vi "set_iterations_per_pixel.vi"(8 "error in (no error)":errorcluster, 10 "iterations per pixel":i32, 11 "FPGAWrapperAN110607Galvo in":refnum<class "FPGAWrapperAN110607Galvo.lvclass">) -> (0 "error out":errorcluster, 3 "FPGAWrapperAN110607Galvo out":refnum<class "FPGAWrapperAN110607Galvo.lvclass">)   [LabVIEW 2010, in "FPGAWrapperAN110607Galvo.lvclass"]
uses:
  FPGAWrapperAN110607Galvo.lvclass
  <vilib>/rvi/interface/nirviReadWriteControl/nirviReadWriteControl.xnode
  FPGA_VI_ref.ctl
  <vilib>/rvi/interface/common/niFpgaNodeNameForErrorReporting.ctl
  <vilib>/rvi/errors/niLvFpgaWhatHappensToTopLevelVI.ctl
  <vilib>/Utility/error.llb/Error Cluster From Error Code.vi
  <vilib>/rvi/errors/niLvFpgaAdjustHostInterfaceError.vi
  NiFpgaLv.dll
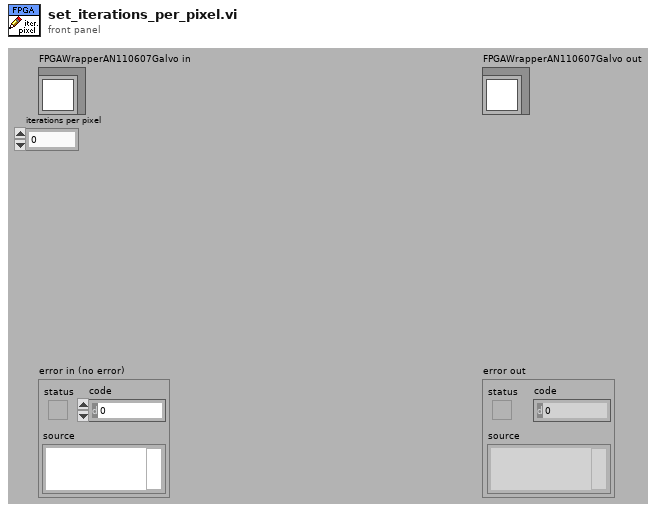
[diagram p1: front panel]
types:
  T1 = typedef "niFpgaNodeNameForErrorReporting.ctl" = enum16{"Open FPGA VI Reference", "Read/Write Control", "Invoke Method: Abort", "Invoke Method: Acknowledge IRQ", "Invoke Method: Download", "Invoke Method: FIFO.Configure", "Invoke Method: FIFO.Read", "Invoke Method: FIFO.Start", "Invoke Method: FIFO.Stop", "Invoke Method: FIFO.Write", "Invoke Method: Reset", "Invoke Method: Run", "Invoke Method: Wait on IRQ", "Close FPGA VI Reference"}
  T2 = typedef "niLvFpgaWhatHappensToTopLevelVI.ctl" = enum16{"top level VI scripted behind XNode", "top level VI inlined behind XNode"}
  T3 = typedef "FPGAWrapperAN110607Galvo.lvclass/FPGA_VI_ref.ctl" = refnum<k20>
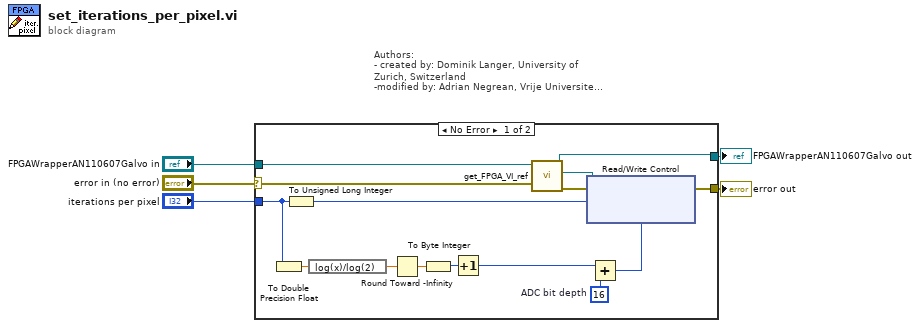
[diagram p0: block diagram]
diagram:
  n1 = case "Authors: \n- created by: Dominik Langer, University of Zurich, Switzerland\n-modified by: Adrian Negrean, Vrije Universiteit Amsterdam" shown="No Error" "error in (no error)" {
    selector: "error in (no error)" -> [w10 w80]
    tunnel: "FPGAWrapperAN110607Galvo in" -> [w11 w81]
    tunnel: [w8 w81] -> w2
    tunnel: [w20 w80] -> w1
    tunnel: "iterations per pixel" -> [w13 _]
    frame No Error {
      w17 = i8 16  # ADC bit depth
      n2 = To Double Precision Float(number=w13) -> (double precision float=w15:dbl)
      n3 = To Unsigned Long Integer(number=w13) -> (unsigned 32bit integer=w19:u32)
      n4 = expression code="log(x)/log(2)"(w15) -> (w14:dbl)
      n5 = Round Toward -Infinity(1:w14) -> (0:w18:dbl)
      n6 = To Byte Integer(number=w18) -> (8bit integer=w16:i8)
      n7 = Increment(x=w16) -> (x+1=w6:i8)
      n8 = call-dynamic "get_FPGA_VI_ref.vi"("error in (no error)"=w10, "FPGAWrapperAN110607Galvo in"=w11) -> ("error out"=w9:errorcluster, "FPGA VI reference"=w12:T3, "FPGAWrapperAN110607Galvo out"=w8:refnum<class "FPGAWrapperAN110607Galvo.lvclass">)  [unwired: 6 in, 1 out]
      n9 = Add(x=w6, y=w17) -> (x+y=w7:i8)
      n10 = xnode "Read/Write Control"("FPGA VI Reference In"=w12, "error in"=w9, "iterations per pixel"=w19, "maximum bit depth"=w7) -> ("error out"=w20:errorcluster)  [unwired: 1 out]
    }
    frame Error {
    }
  }
  "error out" <- w1
  "FPGAWrapperAN110607Galvo out" <- w2
